vi "VecBuilder_1x1Fill.vi"(11 "R0_C0":dbl) -> (3 "output matrix":T1)   [LabVIEW 2019, in "Trajectory_Library.lvlib"]
doc: "Build a 1 x 1 Matrix (vector) from an array of input values.\n\nInputs:\n -- R0_C0 -- Input value\n\nOutputs:\n -- Output Matrix -- Resulting 1 x 1 matrix (vector)"
uses:
  Trajectory_Library.lvlib
  <vilib>/Analysis/Matrix/Datatypes/RealMatrix.ctl
  <vilib>/Analysis/Matrix/NI_Matrix.lvlib
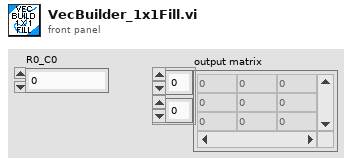
[diagram p1: front panel]
types:
  T1 = typedef "NI_Matrix.lvlib/RealMatrix.ctl" = dbl[][]
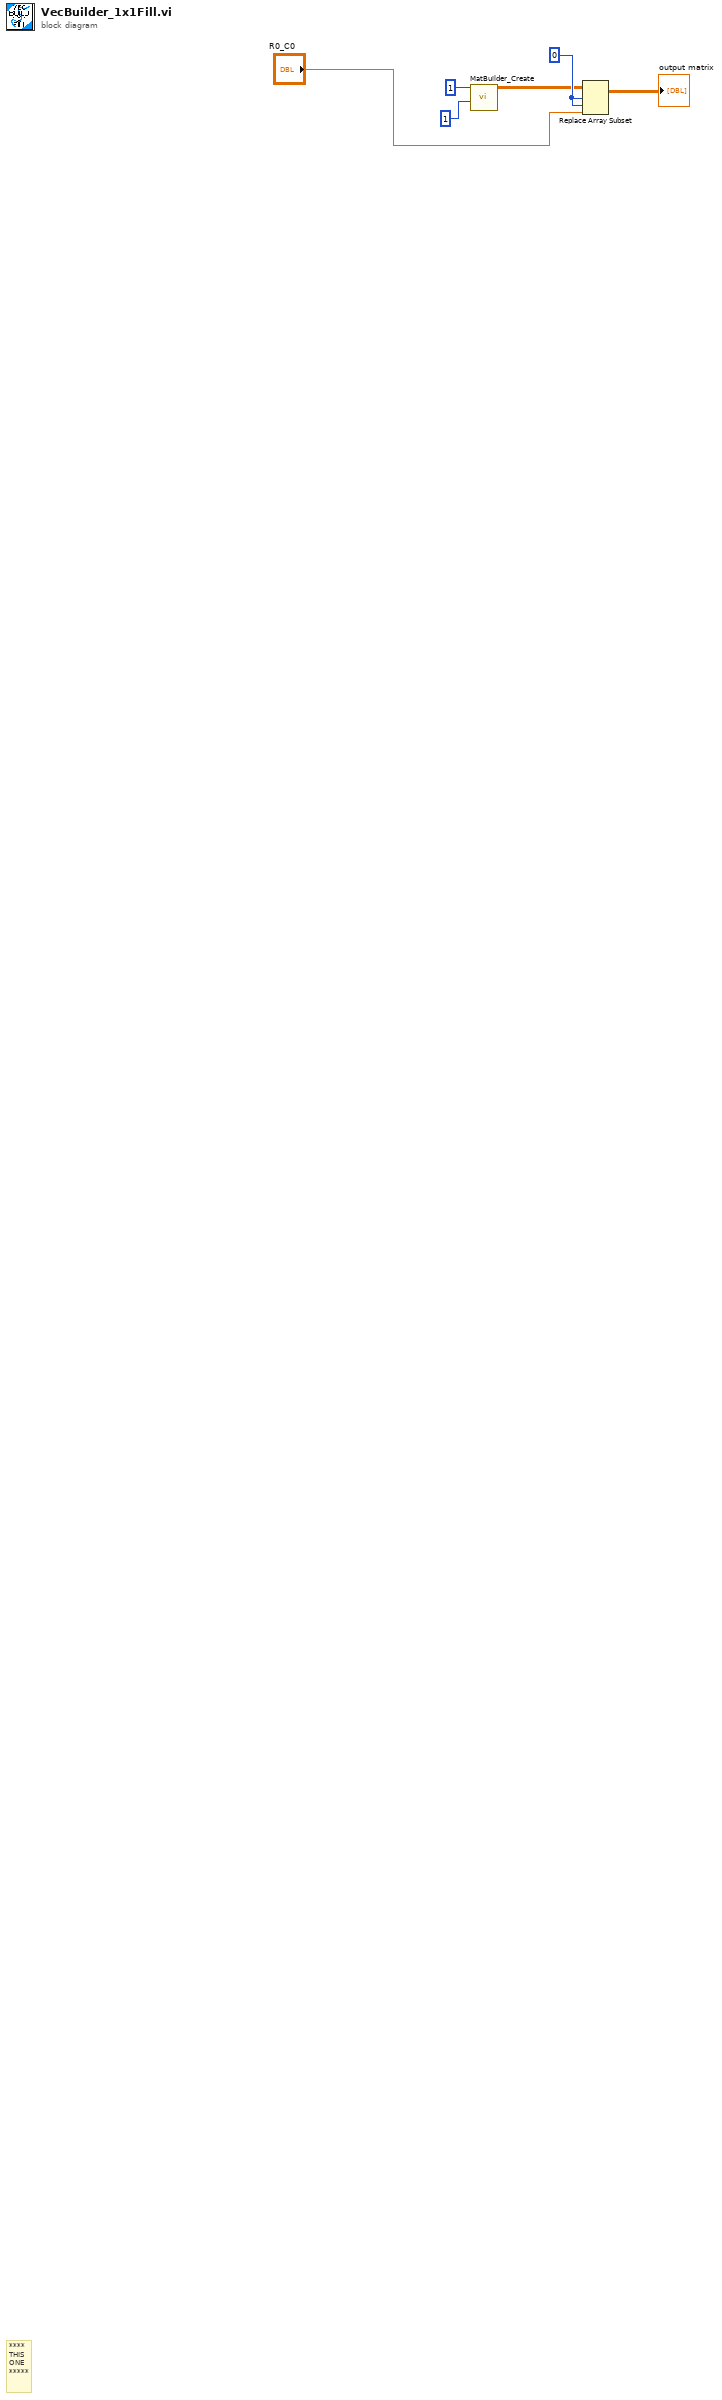
[diagram p0: block diagram]
diagram:
  w6 = 0 ("index (col)")
  # "****\nTHIS\nONE\n*****"
  n1 = call "MatBuilder_Create.vi"("Columns"=1, "Rows"=1) -> ("output matrix"=w1:T1)  [unwired: 9 in]
  n2 = Replace Array Subset(array=w1, new element="R0_C0", index (row)=w6, index (col)=w6) -> (→"output matrix":T1)
